vi "Heartbeat Daemon.vi"(6 "Local Daemon Port":u16, 8 "Error In":errorcluster, 9 "Remote Port":u16, 10 "Target IP":string, 11 "NIVS.Gateway IP Address":string) -> ()   [LabVIEW 2015]
doc: "This host daemon is launched either during the deployment of the heartbeat custom device or, if not detected as running, when the heartbeat service is run. This daemon sends periodic messages to the target, allowing it to know when it's lost communication to the host."
uses:
  <vilib>/NI Veristand/Execution/Workspace/NI_VS Workspace ExecutionAPI.lvlib
panel:
  out "Stopped?":bool
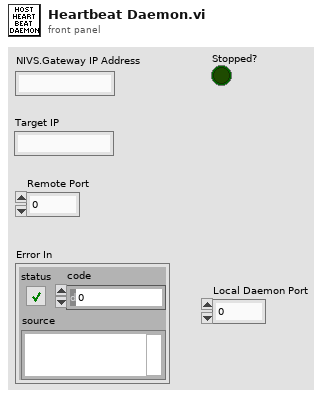
[diagram p1: front panel]
types:
  T1 = typedef "NI_VS Workspace ExecutionAPI.lvlib/WorkspaceAPI.ctl" = refnum<k24>
  T2 = typedef "NI_VS Workspace ExecutionAPI.lvlib/SystemStateEventRef.ctl" = cluster{"CustDatRef":refnum<user-event>, "EvtRef":refnum<k27>, "Target State User Event":refnum<user-event>}
  T3 = typedef "NI_VS Workspace ExecutionAPI.lvlib/SystemStateRegEventRef.ctl" = refnum<event-registration>
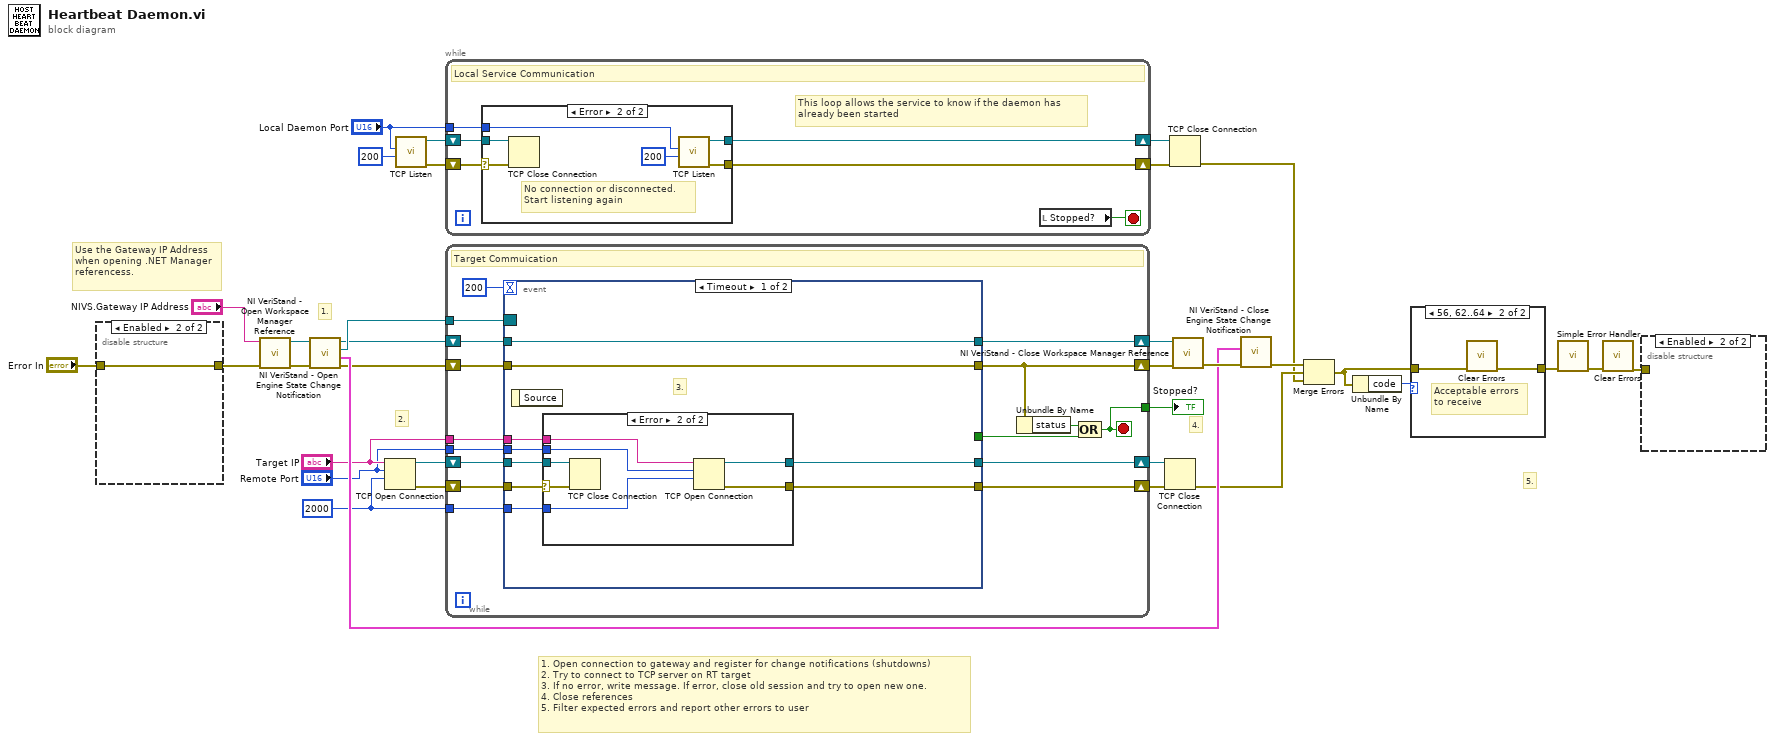
[diagram p0: block diagram]
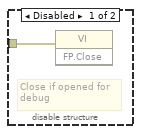
[diagram p4: hidden frame]
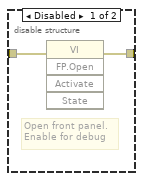
[diagram p5: hidden frame]
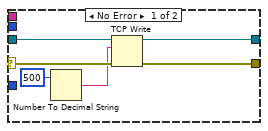
[diagram p6: hidden frame]
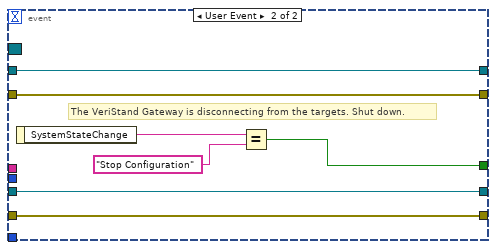
[diagram p7: hidden frame]
diagram:
  w2 = 2000 ("timeout ms (60000)")
  # "1. Open connection to gateway and register for change notifications (shutdowns)\n2. Try to connect to TCP server on RT target\n3. If no error, write message. If error, close old session and try to open new one.\n4. Close references\n5. Filter expected errors and report other errors to user"
  # "5."
  # "4."
  # "2."
  # "1."
  # "Use the Gateway IP Address when opening .NET Manager referencess."
  n1 = disable-structure shown="Enabled" {
    disable-tunnel: [w36 w37] -> w27
    disable-tunnel: "Error In" -> [w35 w37]
    frame Disabled {
      # "Open front panel.\nEnable for debug"
      n2 = invoke class="VI" method="FP.Open"(error in=w35) -> (error out=w36:errorcluster)  [unwired: 4 in, 4 out]
    }
    frame Enabled {
    }
  }
  n3 = call <vilib>:"NI VeriStand - Open Workspace Manager Reference.vi"("error in (no error)"=w27, "Gateway IP Address (\"\": localhost)"="NIVS.Gateway IP Address") -> ("error out"=w30:errorcluster, "WorkspaceManager"=w31:T1)  [unwired: 8 in]
  n4 = call <vilib>:"NI VeriStand - Open Engine State Change Notification.vi"("error in (no error)"=w30, "WorkspaceManager in"=w31) -> ("error out"=w18:errorcluster, "SystemStateRefs"=w28:T2, "SystemChangeEventRef"=w20:T3, "WorkspaceManager out"=w19:T1)  [unwired: 6 in]
  n5 = TCP Open Connection(address="Target IP", remote port or service name="Remote Port", timeout ms (60000)=w2) -> (connection ID=w21:refnum<k5>, error out=w22:errorcluster)  [unwired: 2 in]
  n6 = call <vilib>:"TCP Listen.vi"("timeout ms (wait forever: -1)"=200, "port"="Local Daemon Port") -> ("error out"=w8:errorcluster, "connection ID"=w9:refnum<k5>)  [unwired: 5 in, 3 out]
  n7 = while {
    tunnel: "Local Daemon Port" -> [w41]
    shift-right: [w39] -> w4
    shift-left: w9 -> [w42]
    shift-right: [w40] -> w5
    shift-left: w8 -> [w43]
    stop <- w38 stop-if-true
    # "This loop allows the service to know if the daemon has\nalready been started"
    # "Local Service Communication"
    n8 = case shown="Error" w43 {
      selector: w43 -> [w44 w51]
      tunnel: w42 -> [w45 w50]
      tunnel: [w44 w49] -> w40
      tunnel: [w45 w46] -> w39
      tunnel: w41 -> [_ w47]
      frame No Error {
      }
      frame Error {
        # "No connection or disconnected.\nStart listening again"
        n9 = TCP Close Connection(connection ID=w50, error in (no error)=w51) -> ()  [unwired: 1 in, 2 out]
        n10 = call <vilib>:"TCP Listen.vi"("timeout ms (wait forever: -1)"=200 ("timeout ms (60000)"), "port"=w47) -> ("error out"=w49:errorcluster, "connection ID"=w46:refnum<k5>)  [unwired: 5 in, 3 out]
      }
    }
    n11 = local read "Stopped?"() -> (w38:bool)
  }
  n12 = while {
    tunnel: w20 -> [w67]
    shift-right: [w61] -> w32
    shift-left: w18 -> [w65]
    shift-right: [w64] -> w33
    shift-left: w19 -> [w66]
    shift-right: [w57] -> w24
    shift-left: w22 -> [w58]
    shift-right: [w56] -> w23
    shift-left: w21 -> [w59]
    tunnel: "Target IP" -> [w55]
    tunnel: "Remote Port" -> [w54]
    tunnel: [w53] -> w10
    tunnel: w2 -> [w52]
    stop <- w53 stop-if-true
    # "Target Commuication"
    n13 = event shown="[0] Timeout" {
      selector: w67 -> [_ _]
      dyn-events: _ -> [_ _]
      timeout: 200 -> [_ _]
      tunnel: [_ w92] -> w60
      tunnel: w66 -> [w76 w95]
      tunnel: w65 -> [w75 w96]
      tunnel: [w75 w96] -> w61
      tunnel: [w76 w95] -> w64
      tunnel: w59 -> [w73 w90]
      tunnel: w58 -> [w74 w91]
      tunnel: [w71 w91] -> w57
      tunnel: [w72 w90] -> w56
      tunnel: w55 -> [w70 _]
      tunnel: w54 -> [w69 _]
      tunnel: w52 -> [w68 _]
      event Timeout {
        # "3."
        n14 = event-data() -> ()  [unwired: 1 in, 1 out]
        n15 = case shown="Error" w74 {
          selector: w74 -> [w80 w89]
          tunnel: w73 -> [w81 w88]
          tunnel: [w79 w86] -> w71
          tunnel: [w78 w87] -> w72
          tunnel: w70 -> [_ w84]
          tunnel: w69 -> [_ w85]
          tunnel: w68 -> [_ w83]
          frame No Error {
            n16 = Number To Decimal String(number=u64 500) -> (decimal integer string=w77:string)  [unwired: 1 in]
            n17 = TCP Write(connection ID=w81, data in=w77, error in (no error)=w80) -> (connection ID out=w78:refnum<k5>, error out=w79:errorcluster)  [unwired: 1 in, 1 out]
          }
          frame Error {
            n18 = TCP Close Connection(connection ID=w88, error in (no error)=w89) -> ()  [unwired: 1 in, 2 out]
            n19 = TCP Open Connection(address=w84, remote port or service name=w85, timeout ms (60000)=w83) -> (connection ID=w87:refnum<k5>, error out=w86:errorcluster)  [unwired: 2 in]
          }
        }
      }
      event User Event {
        # "The VeriStand Gateway is disconnecting from the targets. Shut down."
        n20 = event-data() -> ("SystemStateChange"=w94:string)  [unwired: 1 in]
        n21 = Equal?(x=w94, y="Stop Configuration") -> (x = y?=w92:bool)
      }
    }
    n22 = Unbundle By Name(w61) -> ("status"=w62:bool)
    n23 = Compound Arithmetic op=OR(w62, w60) -> (w53:bool)
  }
  "Stopped?" <- w10
  n24 = TCP Close Connection(connection ID=w23, error in (no error)=w24) -> (error out=w16:errorcluster)  [unwired: 1 in, 1 out]
  n25 = TCP Close Connection(connection ID=w4, error in (no error)=w5) -> (error out=w3:errorcluster)  [unwired: 1 in, 1 out]
  n26 = call <vilib>:"NI VeriStand - Close Workspace Manager Reference.vi"("error in (no error)"=w32, "WorkspaceManager"=w33) -> ("error out"=w29:errorcluster)  [unwired: 9 in]
  n27 = call <vilib>:"NI VeriStand - Close Engine State Change Notification.vi"("error in (no error)"=w29, "SystemStateRefs"=w28) -> ("error out"=w17:errorcluster)  [unwired: 9 in]
  n28 = Merge Errors(w17, w16, w3) -> (w15:errorcluster)
  n29 = Unbundle By Name(w15) -> ("code"=w14:i32)
  n30 = case shown="56, 62..64" w14 {
    tunnel: w15 -> [w97 w99]
    tunnel: [w97 w98] -> w12
    frame 0, Default {
    }
    frame 56, 62..64 {
      # "Acceptable errors\nto receive"
      n31 = call <vilib>:"Clear Errors.vi"("error in (no error)"=w99) -> ("error out"=w98:errorcluster)  [unwired: 5 in, 1 out]
    }
  }
  n32 = call <vilib>:"Simple Error Handler.vi"("error in (no error)"=w12) -> ("error out"=w26:errorcluster)  [unwired: 4 in, 4 out]
  n33 = call <vilib>:"Clear Errors.vi"("error in (no error)"=w26) -> ("error out"=w25:errorcluster)  [unwired: 5 in, 1 out]
  n34 = disable-structure shown="Enabled" {
    disable-tunnel: w25 -> [w100 _]
    frame Disabled {
      # "Close if opened for\ndebug"
      n35 = invoke class="VI" method="FP.Close"(error in=w100) -> ()  [unwired: 2 in, 3 out]
    }
    frame Enabled {
    }
  }
